vi "Match Existing Files.vi"(8 "error in (no error)":errorcluster, 9 "incrementor format \" (%d)\"":string=" (%d)", 10 "filename format":string, 11 "directory in":path) -> (0 "error out":errorcluster, 2 "matching filenames":path[](array[path]), 3 "directory out":path)   [LabVIEW 2018, in "Utilities.lvlib"]
uses:
  Utilities.lvlib
  <vilib>/regexp/Match Regular Expression.xnode
panel:
  # "Connector Pane"
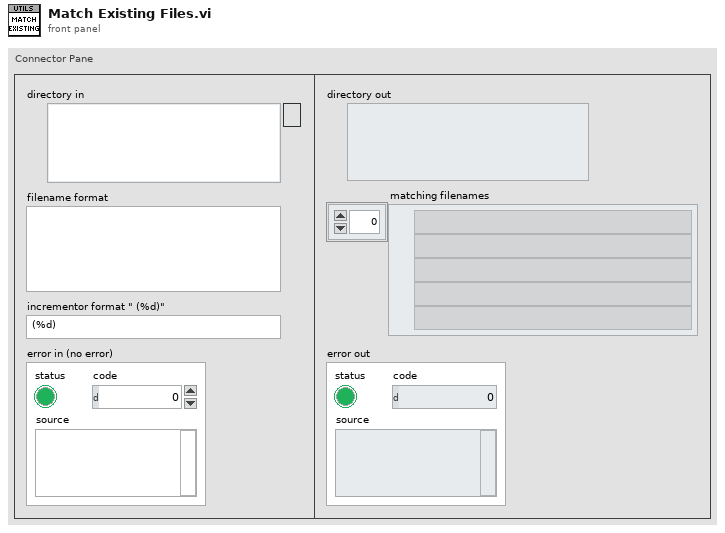
[diagram p1: front panel]
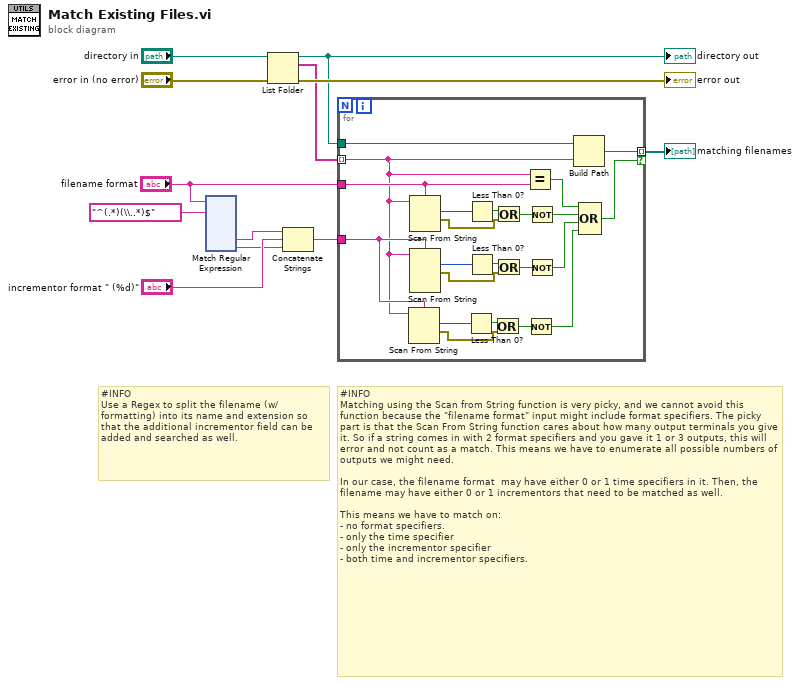
[diagram p0: block diagram]
diagram:
  # "#INFO\nUse a Regex to split the filename (w/formatting) into its name and extension so that the additional incrementor field can be added and searched as well."
  # "#INFO\nMatching using the Scan from String function is very picky, and we cannot avoid this function because the \"filename format\" input might include format specifiers. The picky part is that the Scan From String function cares about how many output terminals you give it. So if a string comes in with 2 format specifiers and you gave it 1 or 3 outputs, this will error and not count as a match. This means we have to enumerate all possible numbers of outputs we might need.\n\nIn our case, the filename format  may have either 0 or 1 time specifiers in it. Then, the filename may have either 0 or 1 incrementors that need to be matched as well.\n\nThis means we have to match on:\n- no format specifiers.\n- only the time specifier\n- only the incrementor specifier\n- both time and incrementor specifiers."
  n1 = xnode "Match Regular Expression"("input string"="filename format", "regular expression"="^(.*)(\\..*)$") -> ("submatch 1"=w6:string, "submatch 2"=w4:string)  [unwired: 4 in, 5 out]
  n2 = List Folder(path="directory in", error in="error in (no error)") -> (path out=w1:path, filenames=w9:string[], error out=→"error out":errorcluster)  [unwired: 2 in, 1 out]
  "directory out" <- w1
  n3 = Concatenate Strings(w6, "incrementor format \" (%d)\"", w4) -> (w2:string)
  n4 = for {
    tunnel: w9 -> [w14] mode=indexing
    tunnel: "filename format" -> [w34]
    tunnel: [w15] -> w8 mode=indexing if=w33
    tunnel: w2 -> [w32]
    tunnel: w1 -> [w13]
    n5 = Scan From String(format string=w32, input string=w14) -> (offset past scan=w21:u32, error out=w20:errorcluster)  [unwired: 4 in, 1 out]
    n6 = Scan From String(format string=w34, input string=w14) -> (offset past scan=w31:u32, error out=w30:errorcluster)  [unwired: 4 in, 1 out]
    n7 = Scan From String(format string=w32, input string=w14) -> (offset past scan=w27:u32, error out=w26:errorcluster)  [unwired: 6 in, 1 out]
    n8 = Less Than 0?(x=w21) -> (x < 0?=w19:bool)
    n9 = Less Than 0?(x=w31) -> (x < 0?=w29:bool)
    n10 = Less Than 0?(x=w27) -> (x < 0?=w25:bool)
    n11 = Or(x=w19, y=w20) -> (x .or. y?=w18:bool)
    n12 = Or(x=w29, y=w30) -> (x .or. y?=w28:bool)
    n13 = Or(x=w25, y=w26) -> (x .or. y?=w24:bool)
    n14 = Equal?(x=w14, y=w34) -> (x = y?=w17:bool)
    n15 = Not(x=w18) -> (.not. x?=w16:bool)
    n16 = Not(x=w28) -> (.not. x?=w22:bool)
    n17 = Not(x=w24) -> (.not. x?=w23:bool)
    n18 = Build Path(base path=w13, name or relative path=w14) -> (appended path=w15:path)
    n19 = Compound Arithmetic op=OR(w17, w22, w23, w16) -> (w33:bool)
  }
  "matching filenames" <- w8
